vi "Measurement-HT.vi"(1 "Ctl Refnum 2":refnum<vi>, 2 "Ctl Refnum":refnum<vi>, 7 "Function (0: Cp-D)":u16(ring) items=["Cp-D", "Cp-Q", "Cp-G", "Cp-Rp", "Cs-D", "Cs-Q", "Cs-Rs", "Lp-D", "Lp-Q", "Lp-G", "Lp-Rp", "Lp-Rdc", "Ls-D", "Ls-Q", "Ls-Rs", "Ls-Rdc", "R-X", "Z-thd", "Z-thr", "G-B", "Y-thd", "Y-thr", "Vdc-Idc"], 8 "error in (no error)":errorcluster, 9 "Byte Stream File Refnum":refnum<file>, 10 "Cluster 2":T1={"结束温度H"=150.0, "变温速率H"=5.0, "簇"={"测试频率"=1000.0, "测试频率 2"=1000.0, "测试频率 3"=1000.0, "测试频率 4"=1000.0}}, 11 "Cluster":T2={"客户仪器地址"="USB0::0x0471::0x2826::QF71600867::INSTR", "高温"="", "高温 2"=""}) -> (0 "error out":errorcluster, 3 "Array":string[][](array[string]))   [LabVIEW 2017]
panel:
  out "修正起始":dbl
  out "修正结束":dbl
  out "内感温":dbl
  out "外感温":dbl
  out "外控温":dbl
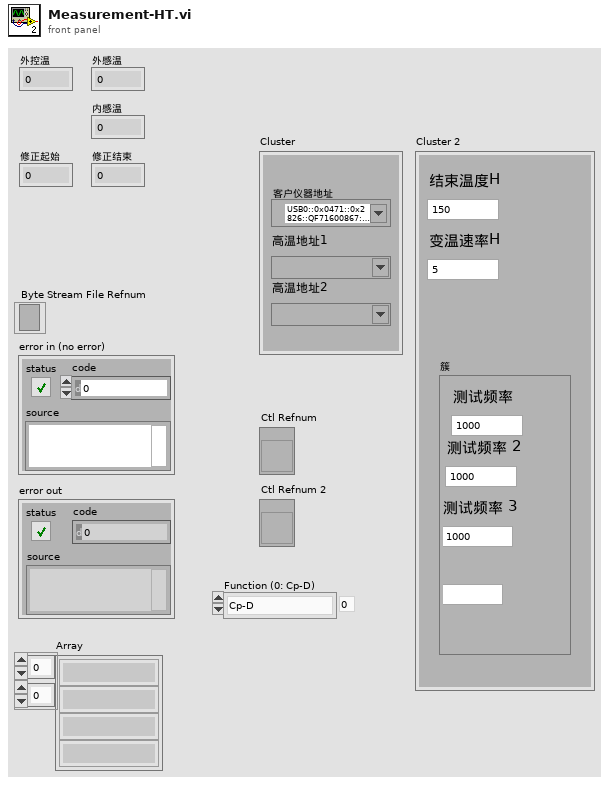
[diagram p1: front panel]
types:
  T1 = cluster{"结束温度H":dbl, "变温速率H":dbl, "簇":cluster{"测试频率":dbl, "测试频率 2":dbl, "测试频率 3":dbl, "测试频率 4":dbl}}
  T2 = cluster{"客户仪器地址":refnum<visa-resource-name>, "高温":refnum<visa-resource-name>, "高温 2":refnum<visa-resource-name>}
  T3 = cluster{"测试频率":dbl, "测试频率 2":dbl, "测试频率 3":dbl, "测试频率 4":dbl}
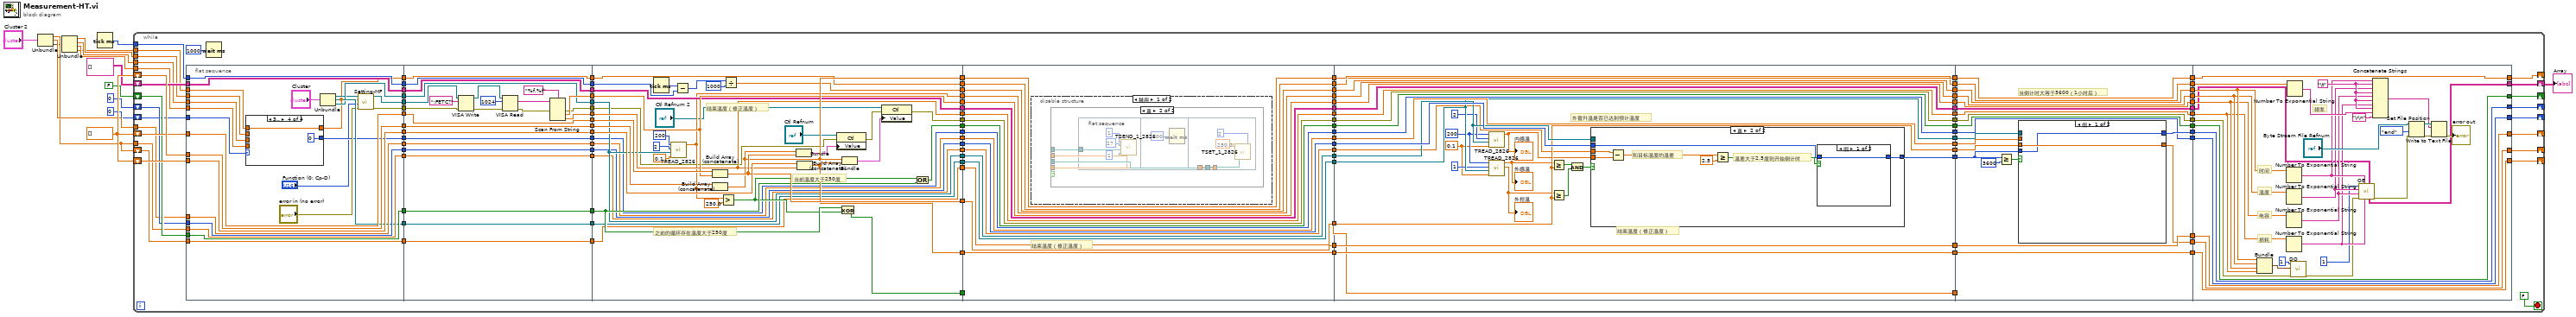
[diagram p0: block diagram]
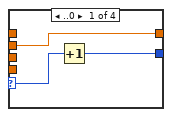
[diagram p2: hidden frame]
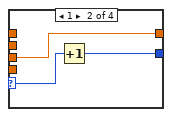
[diagram p3: hidden frame]
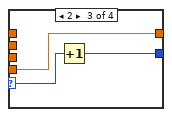
[diagram p4: hidden frame]
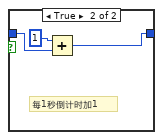
[diagram p8: hidden frame]
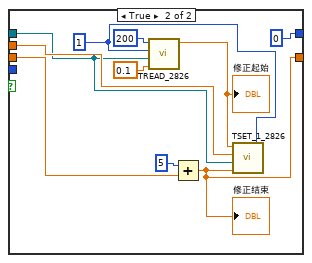
[diagram p9: hidden frame]
diagram:
  w14 = dbl[] []
  n1 = Unbundle("Cluster 2") -> ("结束温度H"=w7:dbl, "变温速率H"=w8:dbl, "簇"=w6:T3)
  n2 = Unbundle(w6) -> ("测试频率"=w4:dbl, "测试频率 2"=w3:dbl, "测试频率 3"=w2:dbl, "测试频率 4"=w1:dbl)
  n3 = Tick Count (ms)() -> (millisecond timer value=w15:u32)
  n4 = while {
    shift-right: [w134] -> _
    shift-left: w14 -> [w141]
    shift-right: [w133] -> _
    shift-left: w14 -> [w140]
    shift-right: [w132] -> _
    shift-left: w14 -> [w139]
    tunnel: w15 -> [w138]
    shift-right: [w136] -> _
    shift-left: FALSE -> [w137]
    shift-right: [w113] -> w11
    shift-left: string[][] [] -> [w110]
    shift-right: [w78] -> _
    shift-left: 0 -> [w103]
    shift-right: [w61] -> _
    shift-left: w7 -> [w56]
    tunnel: w8 -> [w53]
    tunnel: w7 -> [w49]
    shift-right: [w29] -> _
    shift-left: 0 -> [w33]
    tunnel: w4 -> [w32]
    tunnel: w3 -> [w24]
    tunnel: w2 -> [w23]
    tunnel: w1 -> [w22]
    stop <- FALSE stop-if-true
    n5 = flat-sequence {
      tunnel: w49 -> [w157]
      tunnel: w53 -> [w158]
      tunnel: w56 -> [w159]
      tunnel: w103 -> [w160]
      tunnel: w110 -> [w161]
      tunnel: w137 -> [w162]
      tunnel: w138 -> [w163]
      tunnel: w139 -> [w164]
      tunnel: w140 -> [w165]
      tunnel: w141 -> [w166]
      tunnel: [w166] -> w47
      tunnel: [w165] -> w46
      tunnel: [w164] -> w45
      tunnel: [w163] -> w44
      tunnel: [w162] -> w43
      tunnel: [w161] -> w42
      tunnel: [w160] -> w41
      tunnel: [w159] -> w40
      tunnel: [w158] -> w39
      tunnel: [w157] -> w38
      tunnel: [w152] -> w37
      tunnel: [w155] -> w36
      tunnel: [w154] -> w35
      tunnel: [w150] -> w34
      tunnel: w33 -> [w149]
      tunnel: w32 -> [w148]
      tunnel: [w147] -> w31
      tunnel: w24 -> [w146]
      tunnel: w23 -> [w145]
      tunnel: w22 -> [w144]
      tunnel: [w143] -> w16
      tunnel: [w195] -> w131
      tunnel: [w194] -> w130
      tunnel: [w193] -> w129
      tunnel: [w192] -> w128
      tunnel: [w191] -> w127
      tunnel: [w197] -> w126
      tunnel: [w196] -> w125
      tunnel: [w189] -> w114
      tunnel: [w188] -> w111
      tunnel: [w181] -> w109
      tunnel: [w182] -> w107
      tunnel: [w187] -> w104
      tunnel: [w186] -> w57
      tunnel: [w185] -> w54
      tunnel: [w184] -> w48
      tunnel: w47 -> [w195]
      tunnel: w46 -> [w194]
      tunnel: w45 -> [w193]
      tunnel: w44 -> [w192]
      tunnel: w43 -> [w191]
      tunnel: w42 -> [w188]
      tunnel: w41 -> [w187]
      tunnel: w40 -> [w186]
      tunnel: w39 -> [w185]
      tunnel: w38 -> [w184]
      tunnel: w37 -> [w183]
      tunnel: w36 -> [w182]
      tunnel: w35 -> [w181]
      tunnel: w34 -> [w180]
      tunnel: w31 -> [w179]
      tunnel: [w179] -> w30
      tunnel: [w178] -> w17
      tunnel: w16 -> [w178]
      tunnel: [w233] -> w124
      tunnel: w131 -> [w241]
      tunnel: w130 -> [w240]
      tunnel: [w234] -> w123
      tunnel: w129 -> [w239]
      tunnel: [w232] -> w122
      tunnel: w128 -> [w237]
      tunnel: w127 -> [w229]
      tunnel: [w230] -> w121
      tunnel: w126 -> [w226]
      tunnel: [w226] -> w120
      tunnel: w125 -> [w225]
      tunnel: [w225] -> w119
      tunnel: [w224] -> w118
      tunnel: [w217] -> w117
      tunnel: [w223] -> w116
      tunnel: [w211] -> w115
      tunnel: w114 -> [w210]
      tunnel: [w220] -> w112
      tunnel: w111 -> [w220]
      tunnel: w109 -> [w218]
      tunnel: [w219] -> w108
      tunnel: w107 -> [w219]
      tunnel: [w218] -> w106
      tunnel: [w209] -> w105
      tunnel: w104 -> [w209]
      tunnel: [w208] -> w58
      tunnel: w57 -> [w208]
      tunnel: [w207] -> w55
      tunnel: w54 -> [w207]
      tunnel: [w206] -> w50
      tunnel: w48 -> [w206]
      tunnel: w30 -> [w205]
      tunnel: [w205] -> w25
      tunnel: [w204] -> w18
      tunnel: w17 -> [w204]
      tunnel: w124 -> [w259]
      tunnel: [w259] -> w76
      tunnel: w123 -> [w258]
      tunnel: [w258] -> w75
      tunnel: w122 -> [w257]
      tunnel: [w257] -> w74
      tunnel: w121 -> [w256]
      tunnel: [w256] -> w73
      tunnel: w120 -> [w255]
      tunnel: [w255] -> w72
      tunnel: w119 -> [w254]
      tunnel: [w254] -> w71
      tunnel: w118 -> [w253]
      tunnel: [w253] -> w70
      tunnel: w117 -> [w252]
      tunnel: [w252] -> w69
      tunnel: w116 -> [_]
      tunnel: [w251] -> w68
      tunnel: w115 -> [w251]
      tunnel: w112 -> [w250]
      tunnel: [w250] -> w67
      tunnel: w108 -> [w249]
      tunnel: w106 -> [w248]
      tunnel: [w249] -> w66
      tunnel: [w248] -> w65
      tunnel: w105 -> [w247]
      tunnel: [w247] -> w64
      tunnel: [w246] -> w63
      tunnel: [w245] -> w62
      tunnel: w58 -> [w246]
      tunnel: w55 -> [w245]
      tunnel: [w244] -> w51
      tunnel: w50 -> [w244]
      tunnel: [w243] -> w26
      tunnel: w25 -> [w243]
      tunnel: [w242] -> w19
      tunnel: w18 -> [w242]
      tunnel: w76 -> [w302]
      tunnel: [w302] -> w91
      tunnel: w75 -> [w301]
      tunnel: [w301] -> w90
      tunnel: w74 -> [w300]
      tunnel: [w300] -> w89
      tunnel: w73 -> [w299]
      tunnel: [w299] -> w88
      tunnel: w72 -> [w298]
      tunnel: [w298] -> w87
      tunnel: w71 -> [w297]
      tunnel: [w297] -> w86
      tunnel: w70 -> [w296]
      tunnel: [w296] -> w85
      tunnel: w69 -> [w295]
      tunnel: [w295] -> w84
      tunnel: w68 -> [w276]
      tunnel: w67 -> [w294]
      tunnel: [w294] -> w83
      tunnel: [w288] -> w82
      tunnel: w64 -> [w293]
      tunnel: w65 -> [w292]
      tunnel: w63 -> [w287]
      tunnel: [w287] -> w81
      tunnel: [w291] -> w80
      tunnel: w62 -> [w291]
      tunnel: [w290] -> w79
      tunnel: w66 -> [w290]
      tunnel: [w287] -> w59
      tunnel: [w276] -> w52
      tunnel: w51 -> [w283]
      tunnel: [w275] -> w27
      tunnel: w26 -> [w275]
      tunnel: [w274] -> w20
      tunnel: w19 -> [w274]
      tunnel: w91 -> [w334]
      tunnel: [w334] -> w102
      tunnel: w90 -> [w333]
      tunnel: [w333] -> w101
      tunnel: w89 -> [w332]
      tunnel: [w332] -> w100
      tunnel: w88 -> [w331]
      tunnel: [w331] -> w99
      tunnel: w87 -> [w330]
      tunnel: [w330] -> w98
      tunnel: w86 -> [w329]
      tunnel: [w329] -> w97
      tunnel: w85 -> [w328]
      tunnel: [w328] -> w96
      tunnel: w84 -> [w327]
      tunnel: [w327] -> w95
      tunnel: w83 -> [w326]
      tunnel: [w326] -> w94
      tunnel: w82 -> [w322]
      tunnel: [w323] -> w93
      tunnel: w81 -> [_]
      tunnel: w80 -> [w321]
      tunnel: w79 -> [w320]
      tunnel: [w317] -> w77
      tunnel: [w319] -> w60
      tunnel: w59 -> [w318]
      tunnel: w52 -> [w317]
      tunnel: [w316] -> w28
      tunnel: w27 -> [w316]
      tunnel: [w315] -> w21
      tunnel: w20 -> [w315]
      tunnel: w102 -> [w372]
      tunnel: w101 -> [w371]
      tunnel: w100 -> [w370]
      tunnel: w99 -> [w369]
      tunnel: w98 -> [w364]
      tunnel: w97 -> [w363]
      tunnel: w96 -> [w366]
      tunnel: w95 -> [w365]
      tunnel: w94 -> [w358]
      tunnel: [w372] -> w134
      tunnel: [w371] -> w133
      tunnel: [w370] -> w132
      tunnel: [w369] -> w136
      tunnel: [w357] -> w113
      tunnel: [w350] -> w78
      tunnel: w93 -> [w350]
      tunnel: w77 -> [w354]
      tunnel: [w349] -> w61
      tunnel: w60 -> [w349]
      tunnel: [w348] -> w29
      tunnel: w28 -> [w348]
      tunnel: w21 -> [w347]
      frame #0 {
        n6 = case shown="3.." w149 {
          selector: w149 -> [w167 w171 w173 _]
          tunnel: w148 -> [w169 _ _ _]
          tunnel: [w169 w172 w175 w177] -> w143
          tunnel: [w168 w170 w174 0] -> w147
          tunnel: w146 -> [_ w172 _ _]
          tunnel: w145 -> [_ _ w175 _]
          tunnel: w144 -> [_ _ _ w177]
          frame ..0 {
            n7 = Increment(x=w167) -> (x+1=w168:i32)
          }
          frame 1 {
            n8 = Increment(x=w171) -> (x+1=w170:i32)
          }
          frame 2 {
            n9 = Increment(x=w173) -> (x+1=w174:i32)
          }
          frame 3.. {
          }
        }
        n10 = Unbundle("Cluster") -> ("客户仪器地址"=w153:refnum<visa-resource-name>, "高温"=w155:refnum<visa-resource-name>, "高温 2"=w154:refnum<visa-resource-name>)
        n11 = call "Setting-MF.vi"("error in (no error)"="error in (no error)", "Function (0: Cp-D)"="Function (0: Cp-D)", "number"=w143, "VISA resource name"=w153) -> ("error out"=w150:errorcluster, "VISA resource name 2"=w152:refnum<visa-resource-name>)  [unwired: 6 in]
      }
      frame #1 {
        n12 = VISA Write(VISA resource name=w183, write buffer=":FETC?" ("写入缓冲区"), error in (no error)=w180) -> (VISA resource name out=w201:refnum<visa-resource-name>, error out=w202:errorcluster)  [unwired: 1 out]
        n13 = VISA Read(VISA resource name=w201, byte count=u32 1024 ("字节总数"), error in (no error)=w202) -> (read buffer=w199:string, error out=w190:errorcluster)  [unwired: 2 out]
        n14 = Scan From String(format string="%f,%f" ("格式字符串"), input string=w199, error in=w190) -> (error out=w189:errorcluster, output 1=w197:dbl, output 2=w196:dbl)  [unwired: 3 in, 2 out]
      }
      frame #2 {
        # "结束温度（修正温度）"
        # "之前的循环存在温度大于250度"
        # "当前温度大于250度"
        n15 = Tick Count (ms)() -> (millisecond timer value=w238:u32)
        n16 = call "TREAD_2826.vi"("Unknown Param 2"=0.1, "VISA resource name"=w218, "Address No."=i8 2, "Unknown Param"=200) -> ("PV"=w217:dbl)  [unwired: 3 out]
        n17 = Subtract(x=w238, y=w237) -> (x-y=w236:u32)
        n18 = Build Array (concatenate)(w240, w226) -> (w234:dbl[])
        n19 = Build Array (concatenate)(w241, w217) -> (w233:dbl[])
        n20 = Greater?(x=w217, y=250.0) -> (0:w228:bool)
        n21 = Divide(x=w236, y=u32 1000) -> (x/y=w224:dbl)
        n22 = Bundle(w233, w234) -> (w215:cluster{dbl[], dbl[]})  [unwired: 1 in]
        n23 = Build Array (concatenate)(w239, w225) -> (w232:dbl[])
        n24 = property class="Ctl"(reference="Ctl Refnum", error in=w210, "Value"=w215) -> (error out=w212:errorcluster)  [unwired: 1 out]
        n25 = Exclusive Or(1:w228, 2:w229) -> (0:w223:bool)
        n26 = Bundle(w233, w232) -> (w213:cluster{dbl[], dbl[]})  [unwired: 1 in]
        n27 = property class="Ctl"(reference="Ctl Refnum 2", error in=w212, "Value"=w213) -> (error out=w211:errorcluster)  [unwired: 1 out]
        n28 = Or(x=w228, y=w229) -> (x .or. y?=w230:bool)
      }
      frame #3 {
        # "结束温度（修正温度）"
        n29 = disable-structure shown="禁用" {
          frame Disabled {
            n30 = case shown="真" {
              selector: _ -> [_ _]
              tunnel: _ -> [_ w263]
              tunnel: _ -> [_ w262]
              tunnel: _ -> [_ w261]
              tunnel: _ -> [_ w260]
              frame False {
              }
              frame True {
                n31 = flat-sequence {
                  tunnel: w263 -> [w264]
                  tunnel: w262 -> [w271]
                  tunnel: w261 -> [w270]
                  tunnel: w260 -> [w269]
                  frame #0 {
                    n32 = call "TSEND_1_2826.vi"("SettingValue"=i16 1, "VISA resource name"=w264, "No. for reading (Dec.)"=i8 27, "Address No."=i8 1) -> ()  [unwired: 2 out]
                  }
                  frame #1 {
                    n33 = Wait (ms)(milliseconds to wait=u32 200 ("等待时间（毫秒）")) -> ()  [unwired: 1 out]
                  }
                  frame #2 {
                    n34 = call "TSET_1_2826.vi"("Address No."=i8 2, "T-Ending, C"=w270, "VISA resource name"=w271, "cooling/heating rate, C/min"=w269, "T-Starting, C"=250.0) -> ()
                  }
                }
              }
            }
          }
          frame Enabled {
          }
        }
      }
      frame #4 {
        w277 = 0.1
        w278 = 200
        # "结束温度（修正温度）"
        # "外管升温是否已达到预计温度"
        n35 = call "TREAD_2826.vi"("Unknown Param 2"=w277, "VISA resource name"=w292, "Address No."=i8 2, "Unknown Param"=w278) -> ("PV"=w279:dbl)  [unwired: 3 out]
        "内感温" <- w279
        n36 = call "TREAD_2826.vi"("Unknown Param 2"=w277, "VISA resource name"=w290, "Address No."=i8 1, "Unknown Param"=w278) -> ("SV"=w282:dbl, "PV"=w281:dbl)  [unwired: 2 out]
        "外感温" <- w281
        "外控温" <- w282
        n37 = Greater Or Equal?(x=w281, y=w287) -> (x >= y?=w285:bool)
        n38 = Greater Or Equal?(x=w282, y=w287) -> (x >= y?=w284:bool)
        n39 = And(x=w285, y=w284) -> (x .and. y?=w286:bool)
        n40 = case shown="真" w286 {
          tunnel: w293 -> [w303 w310]
          tunnel: [w303 w309] -> w288
          tunnel: w292 -> [_ _]
          tunnel: w283 -> [_ w305]
          tunnel: w279 -> [_ w304]
          frame False {
          }
          frame True {
            # "温差大于2.5度则开始倒计时"
            # "和目标温度的温差"
            n41 = Subtract(x=w305, y=w304) -> (x-y=w308:dbl)
            n42 = Greater Or Equal?(x=w308, y=2.5) -> (x >= y?=w307:bool)
            n43 = case shown="假" w307 {
              tunnel: [w311 w313] -> w309
              tunnel: w310 -> [w311 w312]
              frame False {
              }
              frame True {
                # "每1秒倒计时加1"
                n44 = Add(x=1, y=w312) -> (x+y=w313:i32)
              }
            }
          }
        }
      }
      frame #5 {
        # "当倒计时大等于3600（1小时后）"
        n45 = Greater Or Equal?(x=w322, y=3600) -> (x >= y?=w324:bool)
        n46 = case shown="假" w324 {
          tunnel: [w336 w337] -> w319
          tunnel: w318 -> [w336 w344]
          tunnel: [w335 0] -> w323
          tunnel: w322 -> [w335 _]
          tunnel: w321 -> [_ w341]
          tunnel: w320 -> [_ w340]
          frame False {
          }
          frame True {
            w339 = i8 1 ("Address No.")
            n47 = call "TREAD_2826.vi"("Unknown Param 2"=0.1, "VISA resource name"=w340, "Address No."=w339, "Unknown Param"=200) -> ("PV"=w338:dbl)  [unwired: 3 out]
            "修正起始" <- w338
            n48 = Add(x=5, y=w344) -> (x+y=w337:dbl)
            "修正结束" <- w337
            n49 = call "TSET_1_2826.vi"("Address No."=w339, "T-Ending, C"=w337, "VISA resource name"=w340, "cooling/heating rate, C/min"=w341, "T-Starting, C"=w338) -> ()
          }
        }
      }
      frame #6 {
        w373 = "\t"
        # "频率"
        # "损耗"
        # "电容"
        # "时间"
        # "温度"
        n50 = Bundle(w366, "PV"=w365, w364, w363) -> (w352:cluster{dbl, "PV":dbl, dbl, dbl})  [unwired: 1 in]
        n51 = Number To Exponential String(number=w366) -> (E-format string=w362:string)  [unwired: 3 out]
        n52 = Number To Exponential String(number=w365) -> (E-format string=w361:string)  [unwired: 3 out]
        n53 = Number To Exponential String(number=w364) -> (E-format string=w360:string)  [unwired: 3 out]
        n54 = Number To Exponential String(number=w363) -> (E-format string=w359:string)  [unwired: 3 out]
        n55 = Number To Exponential String(number=w347) -> (E-format string=w375:string)  [unwired: 3 out]
        n56 = call "DO.vi"("error in (no error)"=w354, "数据输出"=w352, "功能编号"=1) -> ("error out"=w353:errorcluster)  [unwired: 8 in]
        n57 = call "OE.vi"("Array"=w358, "String 4"=w359, "String"=w362, "error in (no error)"=w353, "String 3"=w360, "String 2"=w361, "Numeric"=1) -> ("error out"=w355:errorcluster, "Array 2"=w357:string[][])  [unwired: 2 in, 1 out]
        n58 = Concatenate Strings(w362, w373, w361, w373, w360, w373, w359, w373, w375, "\r\n") -> (w377:string)
        n59 = Set File Position(refnum="Byte Stream File Refnum", from (0:start)=enum16{"start", "end", "current"}."end" ("自（0:起始）"), error in=w355) -> (refnum out=w379:refnum<file>, error out=w376:errorcluster)  [unwired: 1 out]
        n60 = Write to Text File(file (use dialog)=w379, text=w377, error in=w376) -> (error out=→"error out":errorcluster)  [unwired: 3 out]
      }
    }
    n61 = Wait (ms)(milliseconds to wait=1000) -> ()  [unwired: 1 out]
  }
  "Array" <- w11
